vi "RunOperation.vi"(10 "Inputs":string[](array[string]), 11 "SetConditionalSymbol in":refnum<class "SetConditionalSymbol.lvclass">) -> (1 "Output/Failure":string, 2 "CLI Process Return Code":i32, 3 "SetConditionalSymbol out":refnum<class "SetConditionalSymbol.lvclass">)   [LabVIEW 2023, in "SetConditionalSymbol.lvclass"]
doc: "Entry point for LabVIEWCLI."
uses:
  SetConditionalSymbol.lvclass
  SetConditionalSymbol.lvclass/SetConditionalSymbol.ctl
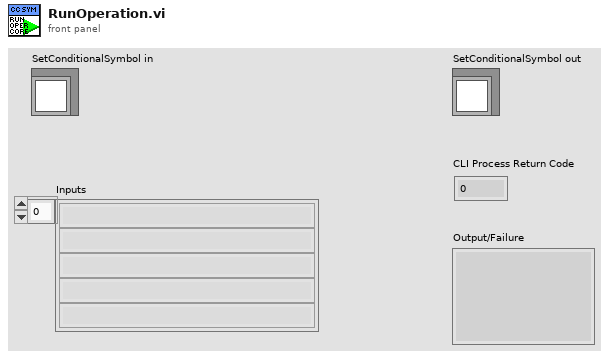
[diagram p1: front panel]
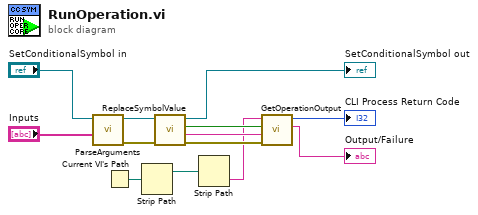
[diagram p0: block diagram]
diagram:
  n1 = call "ParseArguments.vi"("Inputs"="Inputs", "SetConditionalSymbol in"="SetConditionalSymbol in") -> ("error out"=w10:errorcluster, "SetConditionalSymbol out"=w11:refnum<class "SetConditionalSymbol.lvclass">)  [unwired: 8 in]
  n2 = Current VI's Path() -> (path=w5:path)
  n3 = Strip Path(path=w5) -> (stripped path=w4:path)  [unwired: 1 out]
  n4 = call "ReplaceSymbolValue.vi"("error in (no error)"=w10, "SetConditionalSymbol in"=w11) -> ("error out"=w7:errorcluster, "Output/Failure"=w6:string, "Success?"=w8:bool, "SetConditionalSymbol out"=→"SetConditionalSymbol out":refnum<class "SetConditionalSymbol.lvclass">)  [unwired: 6 in]
  n5 = Strip Path(path=w4) -> (name=w3:string)  [unwired: 1 out]
  n6 = call "GetOperationOutput.vi"("error in (no error)"=w7, "Operation Output/Error In"=w6, "Operation succeeded?"=w8, "Operation Name"=w3) -> ("Operation Output/Error Out"=→"Output/Failure":string, "CLI Process Return Code"=→"CLI Process Return Code":i32)  [unwired: 6 in]
